vi "GFITS_exec_autocmds.vi"(0 "commands2exec":string) -> ()   [LabVIEW 2016]
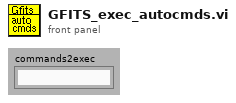
[diagram p1: front panel]
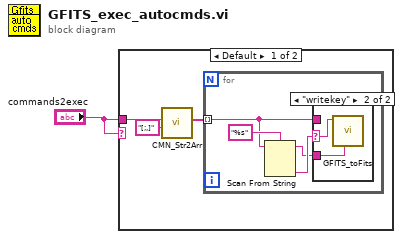
[diagram p0: block diagram]
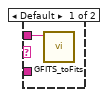
[diagram p2: hidden frame]
diagram:
  n1 = case shown="Default" "commands2exec" {
    tunnel: "commands2exec" -> [w4 _]
    frame Default {
      n2 = call "CMN_Str2Arr.vi"("separator"="[;,]", "string in"=w4) -> ("Array out"=w3:string[])  [unwired: 2 in, 7 out]
      n3 = for {
        tunnel: w3 -> [w6] mode=indexing
        n4 = Scan From String(format string="%s", input string=w6) -> (remaining string=w5:string, output 1=w7:string)  [unwired: 2 in, 3 out]
        n5 = case shown="\"writekey\"" w7 {
          selector: w7 -> [_ w10]
          tunnel: w6 -> [w9 _]
          tunnel: w5 -> [_ w11]
          frame Default {
            n6 = call "GFITS_toFits.vi"("command"=w9) -> ()  [unwired: 8 in, 3 out]
          }
          frame "writekey" {
            n7 = call "GFITS_toFits.vi"("key"=w11, "command"=w10) -> ()  [unwired: 7 in, 3 out]
          }
        }
      }
    }
    frame "", " ", "none" {
    }
  }
